vi "String Field To Integer.vi"(8 "error in (no error)":errorcluster, 11 "Sudoku Class in":refnum<class "Sudoku Class.lvclass">) -> (0 "error out":errorcluster, 2 "Sudoku Int":u8[][](array[numeric]), 3 "Sudoku Class out":refnum<class "Sudoku Class.lvclass">)   [LabVIEW 2015, in "Sudoku Library.lvlib" / "Sudoku Class.lvclass"]
doc: "Created IvanLis by LabVIEW Portal\nProfile: http://labviewportal.org/memberlist.php?mode=viewprofile&u=987\neMail: IvanLisanov@gMail.com\nTelegram: https://t.me/IvanLis"
uses:
  Sudoku Class.lvclass
  Sudoku Class.lvclass/Sudoku Class.ctl
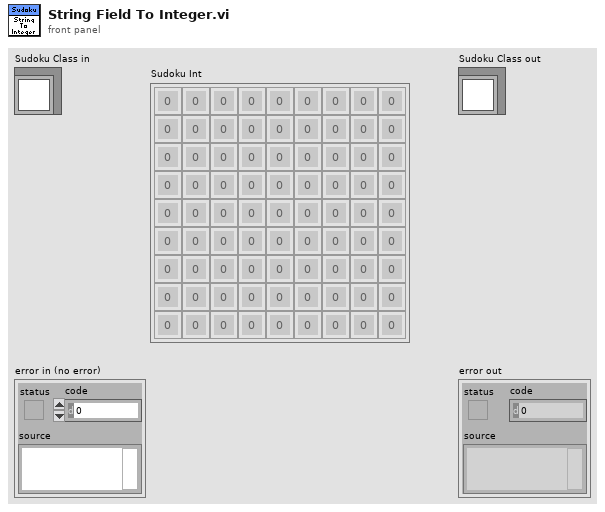
[diagram p1: front panel]
types:
  T1 = typedef "Sudoku Library.lvlib/Sudoku String.ctl" = string[][]
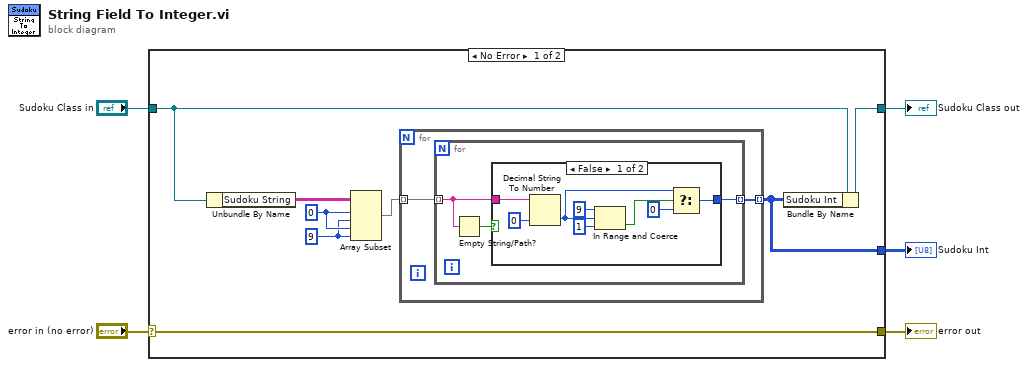
[diagram p0: block diagram]
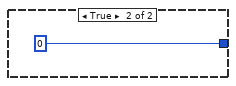
[diagram p2: hidden frame]
diagram:
  n1 = case shown="No Error" "error in (no error)" {
    selector: "error in (no error)" -> [w11 w29]
    tunnel: [w11 w29] -> w4
    tunnel: [w12 w28] -> w2
    tunnel: "Sudoku Class in" -> [w13 w28]
    tunnel: [w10 _] -> w1
    frame No Error {
      w8 = 9 ("length")
      w9 = 0 ("index")
      n2 = Unbundle By Name(w13) -> ("Sudoku String"=w6:T1)
      n3 = Array Subset(array=w6, index (row)=w9, length (row)=w8, index (col)=w9, length (col)=w8) -> (w7:T1)
      n4 = for {
        tunnel: w7 -> [w15] mode=indexing
        tunnel: [w14] -> w10 mode=indexing
        n5 = for {
          tunnel: w15 -> [w16] mode=indexing
          tunnel: [w17] -> w14 mode=indexing
          n6 = Empty String/Path?(string/path=w16) -> (empty?=w18:bool)
          n7 = case shown="False" w18 {
            tunnel: [w22 u8 0] -> w17
            tunnel: w16 -> [w26 _]
            frame False {
              n8 = Decimal String To Number(string=w26, default (0L)=u8 0 ("default (0 I32)")) -> (number=w20:u8)  [unwired: 1 in, 1 out]
              n9 = In Range and Coerce(upper limit=u8 9, x=w20, lower limit=u8 1) -> (In Range?=w21:bool)  [unwired: 1 out]
              n10 = Select(t=w20, s=w21, f=u8 0) -> (s? t:f=w22:u8)
            }
            frame True {
            }
          }
        }
      }
      n11 = Bundle By Name(cluster=w13, "Sudoku Int"=w10) -> (w12:refnum<class "Sudoku Class.lvclass">)
    }
    frame Error {
    }
  }
  "error out" <- w4
  "Sudoku Class out" <- w2
  "Sudoku Int" <- w1
